vi "Get MIDI bytes.vi"   [LabVIEW 2015]
uses:
  <vilib>/rvi/Emulation/niFpgaGetClockAttributes.vi
  <vilib>/rvi/Emulation/niFpgaSctlEmulationGetInTimedLoop.vi
  <vilib>/rvi/Emulation/niFpgaEmulationReportErrorSimple.vi
  MIDI/Controls/Stop.vi
  <vilib>/rvi/eio/common/nirviEmuTemplateMethod_errors.vi
  <vilib>/rvi/Emulation/niFpgaCriticalErrorInLSC.vi
  <vilib>/rvi/interface/RandomDataEmulation/niFpgaRandomDataHandleErrors.vi
  <vilib>/eio/EIONode/EIONode.xnode
  <vilib>/rvi/DataTransferAndStorage/Container/XNode/niFpgaContainer.xnode
  <vilib>/rvi/interface/RandomDataEmulation/nirviRandomDataFpgaReadWriteTemplate.vi
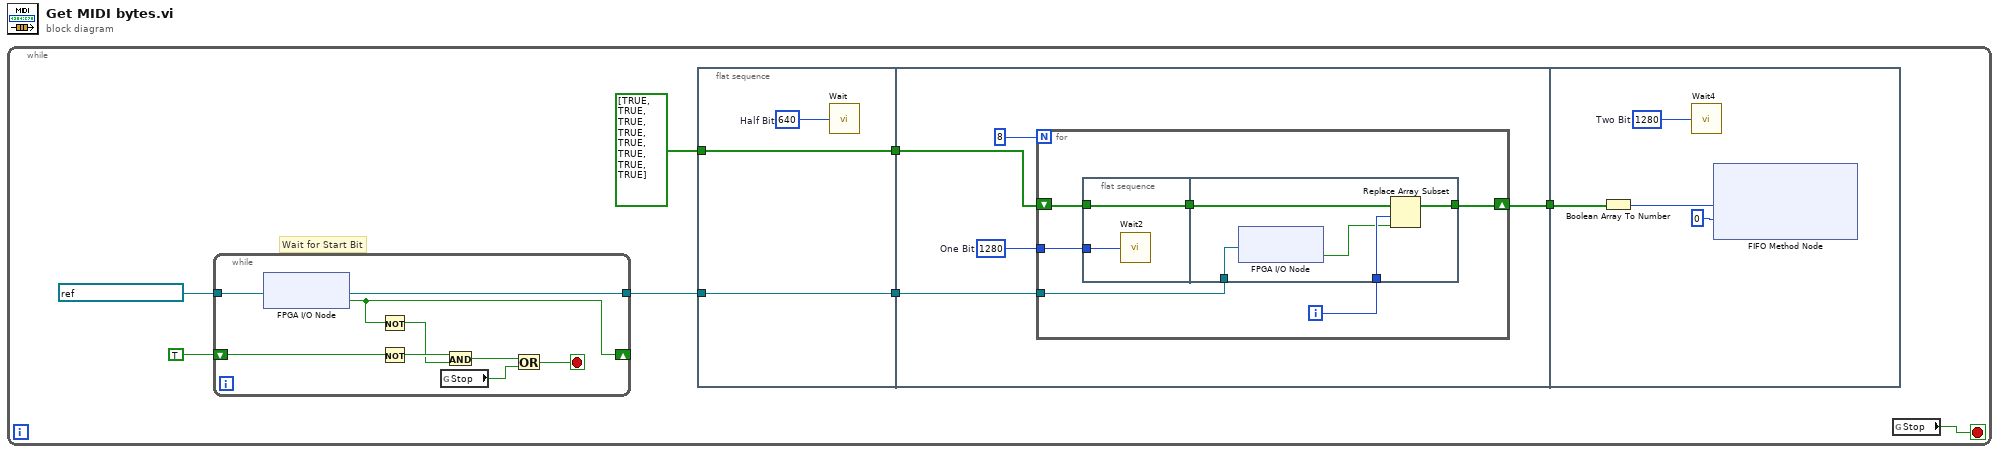
[diagram p0: block diagram]
diagram:
  n1 = while {
    stop <- w6 stop-if-true
    # "Wait for Start Bit"
    n2 = while {
      shift-right: [w35] -> _
      shift-left: TRUE -> [w42]
      tunnel: refnum<k21> "ConnectorA/DIO10" ("Receive") -> [w38]
      tunnel: [w34] -> w3
      stop <- w39 stop-if-true
      n3 = xnode "FPGA I/O Node"("FPGA I/O In"=w38) -> ("I/O Item"=w35:bool, "FPGA I/O Out"=w34:refnum<k21>)
      n4 = Not(x=w35) -> (.not. x?=w36:bool)
      n5 = Not(x=w42) -> (.not. x?=w41:bool)
      n6 = global read "Stop.vi" "Stop"() -> (w37:bool)
      n7 = And(x=w41, y=w36) -> (x .and. y?=w40:bool)
      n8 = Or(x=w40, y=w37) -> (x .or. y?=w39:bool)
    }
    n9 = flat-sequence {
      tunnel: [w11] -> w5
      tunnel: bool[] [TRUE, TRUE, TRUE, TRUE, TRUE, TRUE, TRUE, TRUE] -> [w11]
      tunnel: w3 -> [w9]
      tunnel: [w9] -> w2
      tunnel: w5 -> [w16]
      tunnel: w2 -> [w13]
      tunnel: [w12] -> w1
      tunnel: w1 -> [w32]
      frame #0 {
        w10 = u32 640  # Half Bit
        n10 = call "Wait"("Count(Ticks)"=w10) -> ()  [unwired: 1 out]
      }
      frame #1 {
        w14 = u32 1280  # One Bit
        n11 = for {
          N: 8 ("data bits (8)") -> [_]
          shift-right: [w19] -> w12
          shift-left: w16 -> [w22]
          tunnel: w14 -> [w20]
          tunnel: w13 -> [w18]
          i -> [w17]
          n12 = flat-sequence {
            tunnel: w22 -> [w24]
            tunnel: [w24] -> w21
            tunnel: w20 -> [w23]
            tunnel: w21 -> [w29]
            tunnel: [w28] -> w19
            tunnel: w18 -> [w27]
            tunnel: w17 -> [w26]
            frame #0 {
              n13 = call "Wait2"("Count(Ticks)"=w23) -> ()  [unwired: 1 out]
            }
            frame #1 {
              n14 = xnode "FPGA I/O Node"("FPGA I/O In"=w27) -> ("I/O Item"=w25:bool)  [unwired: 1 out]
              n15 = Replace Array Subset(array=w29, new element=w25, index=w26) -> (w28:bool[])
            }
          }
        }
      }
      frame #2 {
        w33 = u32 1280  # Two Bit
        n16 = Boolean Array To Number(Boolean array=w32) -> (number=w31:u8)
        n17 = call "Wait4"("Count(Ticks)"=w33) -> ()  [unwired: 1 out]
        n18 = xnode ("FIFO Method Node")("Element"=w31, "Timeout"=0) -> ()  [unwired: 1 in, 2 out]
      }
    }
    n19 = global read "Stop.vi" "Stop"() -> (w6:bool)
  }
